vi "Dispense FN - ON - Setpoints - Dynamic (SubVI).vi"(0 "Enable Dynamic Setpoint?":bool, 1 "Measured Mass (g)":dbl, 2 "Static Setpoint (g)":dbl, 3 "% of Setpoint per Spray":dbl[](array[numeric]), 4 "State Change?":bool, 5 "Main Case Change?":bool, 7 "Dynamic Mass Factor (g)":dbl) -> (14 "Dynamic Setpoint (g)":dbl)   [LabVIEW 2012]
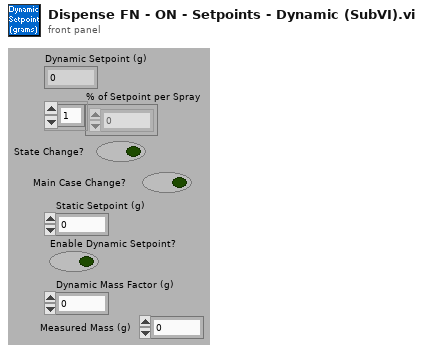
[diagram p1: front panel]
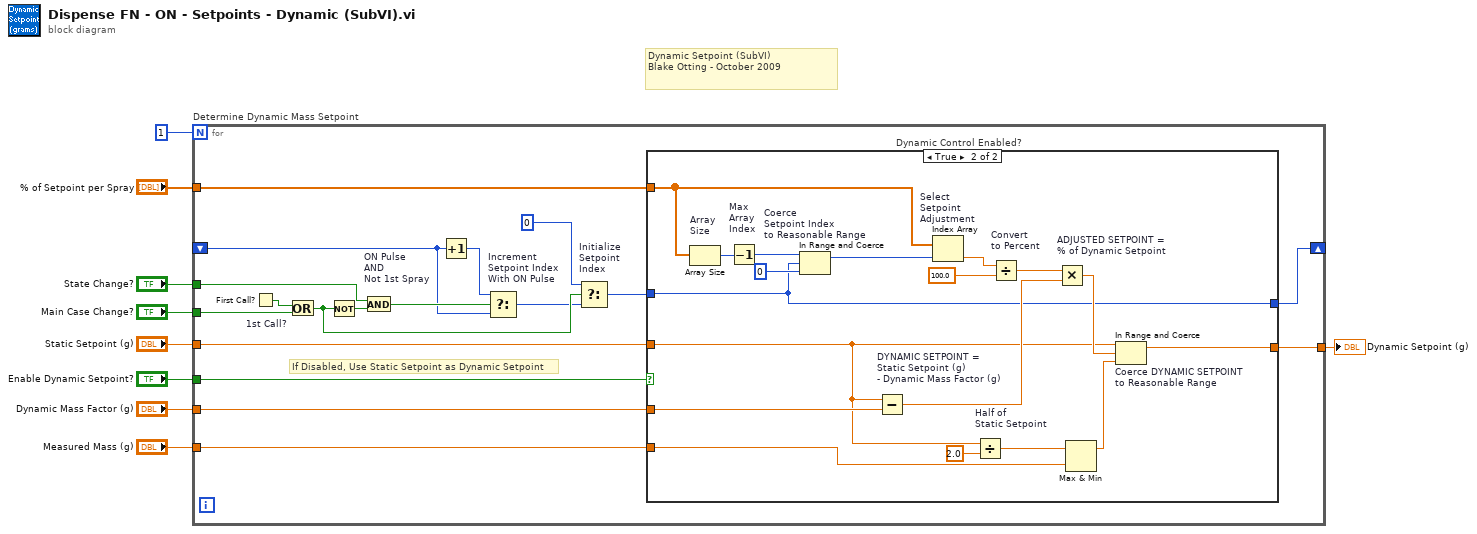
[diagram p0: block diagram]
diagram:
  # "Dynamic Setpoint (SubVI)\nBlake Otting - October 2009"
  n1 = for "Determine Dynamic Mass Setpoint" {
    N: 1 -> [_]
    tunnel: "Measured Mass (g)" -> [w25]
    tunnel: "Main Case Change?" -> [w20]
    shift-right: [w26] -> _
    shift-left: _ -> [w10]
    tunnel: "State Change?" -> [w18]
    tunnel: "Static Setpoint (g)" -> [w17]
    tunnel: "Dynamic Mass Factor (g)" -> [w16]
    tunnel: "% of Setpoint per Spray" -> [w15]
    tunnel: "Enable Dynamic Setpoint?" -> [w14]
    tunnel: [w13] -> w9
    # "If Disabled, Use Static Setpoint as Dynamic Setpoint"
    n2 = First Call? "1st Call?"() -> (First Call?: T/F=w19:bool)
    n3 = Or(x=w19, y=w20) -> (x .or. y?=w21:bool)
    n4 = Not(x=w21) -> (.not. x?=w22:bool)
    n5 = And "ON Pulse\nAND\nNot 1st Spray"(x=w18, y=w22) -> (x .and. y?=w23:bool)
    n6 = Increment(x=w10) -> (x+1=w24:i32)
    n7 = Select "Increment\nSetpoint Index\nWith ON Pulse"(t=w24, s=w23, f=w10) -> (s? t:f=w11:i32)
    n8 = Select "Initialize\nSetpoint\nIndex"(t=0, s=w21, f=w11) -> (s? t:f=w12:i32)
    n9 = case "Dynamic Control Enabled?" shown="True" w14 {
      tunnel: w17 -> [w28 w34]
      tunnel: [w28 w46] -> w13
      tunnel: w12 -> [w29 w35]
      tunnel: [w29 w35] -> w26
      tunnel: w15 -> [_ w40]
      tunnel: w25 -> [_ w32]
      tunnel: w16 -> [_ w44]
      frame False {
        # "Use Static Setpoint\nIF \nDynamic Setpoint is Disabled"
      }
      frame True {
        n10 = Array Size "Array\nSize"(array=w40) -> (size(s)=w39:i32)
        n11 = Decrement "Max\nArray\nIndex"(x=w39) -> (x-1=w38:i32)
        n12 = In Range and Coerce "Coerce \nSetpoint Index\nto Reasonable Range"(upper limit=w38, x=w35, lower limit=0) -> (coerced(x)=w36:i32)  [unwired: 1 out]
        n13 = Subtract "DYNAMIC SETPOINT =\nStatic Setpoint (g)\n- Dynamic Mass Factor (g)"(x=w34, y=w44) -> (x-y=w43:dbl)
        n14 = Index Array "Select\nSetpoint\nAdjustment"(array=w40, index=w36) -> (element=w47:dbl)
        n15 = Divide "Half of\nStatic Setpoint"(x=w34, y=2.0) -> (x/y=w31:dbl)
        n16 = Divide "Convert\nto Percent"(x=w47, y=100.0) -> (x/y=w42:dbl)
        n17 = Multiply "ADJUSTED SETPOINT = \n% of Dynamic Setpoint"(x=w42, y=w43) -> (x*y=w41:dbl)
        n18 = Max & Min(x=w31, y=w32) -> (max(x,y)=w30:dbl)  [unwired: 1 out]
        n19 = In Range and Coerce "Coerce DYNAMIC SETPOINT\nto Reasonable Range"(upper limit=w34, x=w41, lower limit=w30) -> (coerced(x)=w46:dbl)  [unwired: 1 out]
      }
    }
  }
  "Dynamic Setpoint (g)" <- w9
